vi "Hysteresis-PhaseDelayCorrection.vi"(9 "size":i32, 10 "FWD/BWD":cluster{"bwd ":i32[], "fwd":i32[]}) -> (1 "pixel to delete":dbl, 2 "Corrected":T1)   [LabVIEW 2016]
uses:
  <vilib>/Analysis/NI_AALPro.lvlib
panel:
  out "fwd=f(bwd)":dbl
  out "bwd=f(fwd)":dbl
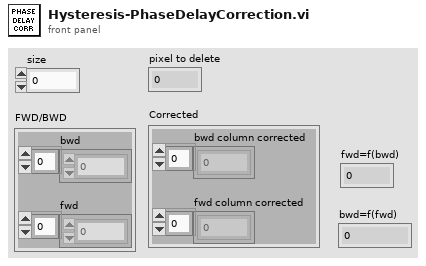
[diagram p1: front panel]
types:
  T1 = cluster{"bwd column corrected":dbl[], "fwd column corrected":dbl[]}
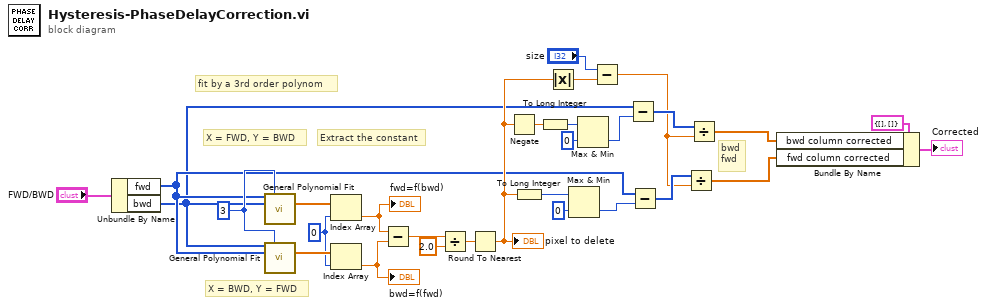
[diagram p0: block diagram]
diagram:
  w3 = 0 ("index")
  w4 = 3 ("polynomial order")
  # "Extract the constant"
  # "fit by a 3rd order polynom"
  # "X = FWD, Y = BWD"
  # "X = BWD, Y = FWD"
  # "bwd\nfwd"
  n1 = Unbundle By Name("FWD/BWD") -> ("fwd"=w2:i32[], "bwd"=w1:i32[])
  n2 = call <vilib>:"General Polynomial Fit.vi"("Y"=w2, "polynomial order"=w4, "X"=w1) -> ("Polynomial Coefficients"=w11:dbl[])  [unwired: 9 in, 3 out]
  n3 = call <vilib>:"General Polynomial Fit.vi"("Y"=w1, "polynomial order"=w4, "X"=w2) -> ("Polynomial Coefficients"=w10:dbl[])  [unwired: 9 in, 3 out]
  n4 = Index Array(array=w11, index=w3) -> (element=w12:dbl)
  "fwd=f(bwd)" <- w12
  n5 = Index Array(array=w10, index=w3) -> (element=w13:dbl)
  "bwd=f(fwd)" <- w13
  n6 = Subtract(x=w12, y=w13) -> (x-y=w14:dbl)
  n7 = Divide(x=w14, y=2.0) -> (x/y=w16:dbl)
  n8 = Round To Nearest(number=w16) -> (nearest integer value=w28:dbl)
  "pixel to delete" <- w28
  n9 = Negate(x=w28) -> (-x=w26:dbl)
  n10 = To Long Integer(number=w28) -> (32bit integer=w21:i32)
  n11 = To Long Integer(number=w26) -> (32bit integer=w20:i32)
  n12 = Absolute Value(x=w28) -> (abs(x)=w17:dbl)
  n13 = Max & Min(x=w21, y=0) -> (min(x,y)=w23:i32)  [unwired: 1 out]
  n14 = Max & Min(x=w20, y=0) -> (min(x,y)=w27:i32)  [unwired: 1 out]
  n15 = Subtract(x="size", y=w17) -> (x-y=w18:dbl)
  n16 = Subtract(x=w1, y=w27) -> (x-y=w25:i32[])
  n17 = Subtract(x=w2, y=w23) -> (x-y=w24:i32[])
  n18 = Divide(x=w24, y=w18) -> (x/y=w5:dbl[])
  n19 = Divide(x=w25, y=w18) -> (x/y=w6:dbl[])
  n20 = Bundle By Name(cluster=T1 {"bwd column corrected"=[], "fwd column corrected"=[]} ("Corrected"), "bwd column corrected"=w6, "fwd column corrected"=w5) -> (→"Corrected":T1)
